vi "Deney 1.vi"() -> ()   [LabVIEW 2018]
panel:
  in  "T":dbl(knob) scale=0.0..100.0
  out "Thermometer":dbl(knob) scale=0.0..100.0
  in  "B":dbl(slide) scale=0.0..212.0
  in  "A":dbl(slide) scale=0.0..100.0
  out "HIGH":bool
  out "LOW":bool
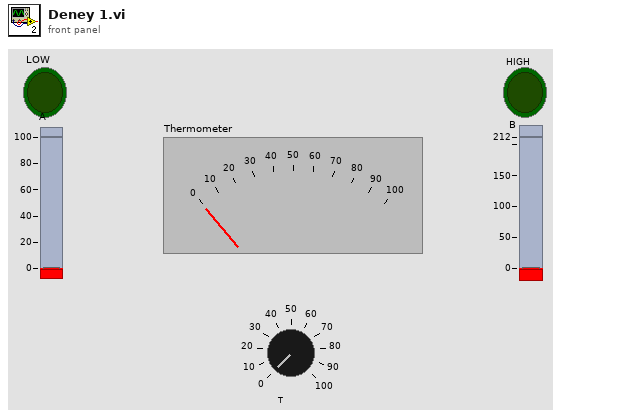
[diagram p1: front panel]
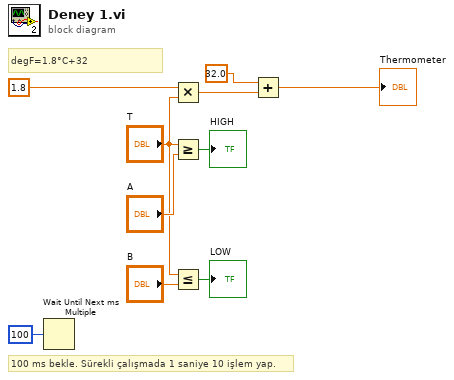
[diagram p0: block diagram]
diagram:
  # "100 ms bekle. Sürekli çalışmada 1 saniye 10 işlem yap."
  # "degF=1.8°C+32"
  n1 = Wait Until Next ms Multiple(millisecond multiple=100) -> ()  [unwired: 1 out]
  n2 = Multiply(x=1.8, y="T") -> (x*y=w3:dbl)
  n3 = Greater Or Equal?(x="T", y="A") -> (x >= y?=→"HIGH":bool)
  n4 = Less Or Equal?(x="T", y="B") -> (x <= y?=→"LOW":bool)
  n5 = Add(x=32.0, y=w3) -> (x+y=→"Thermometer":dbl)
